vi "XNET Database Export.vi"(0 "cluster in":refnum<k21>, 5 "filepath":path, 11 "error in (no error)":errorcluster) -> (4 "cluster out":refnum<k21>, 15 "error out":errorcluster)   [LabVIEW 2018]
doc: "Exports the cluster to a file in a specific format (.dbc for a CAN cluster, .ldf for a LIN cluster)."
uses:
  nixlvapi.dll
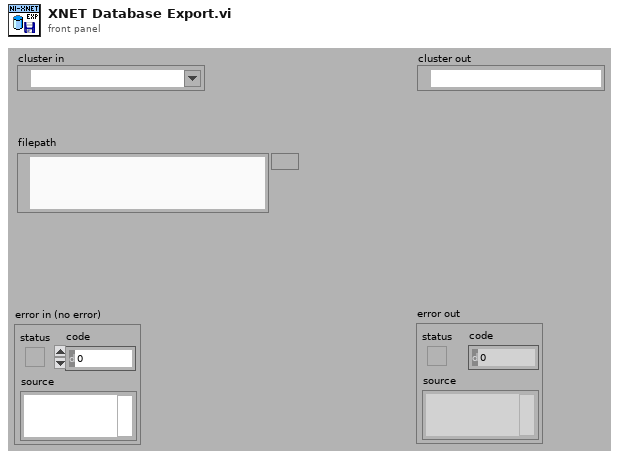
[diagram p1: front panel]
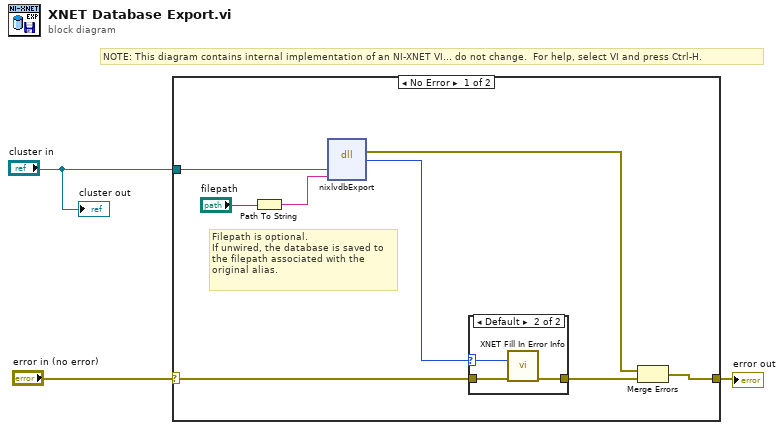
[diagram p0: block diagram]
diagram:
  # "NOTE: This diagram contains internal implementation of an NI-XNET VI... do not change.  For help, select VI and press Ctrl-H."
  n1 = case shown="No Error" "error in (no error)" {
    selector: "error in (no error)" -> [w8 w16]
    tunnel: "cluster in" -> [w11 _]
    tunnel: [w5 w16] -> w3
    frame No Error {
      # "Filepath is optional.\nIf unwired, the database is saved to\nthe filepath associated with the\noriginal alias."
      n2 = Path To String(path="filepath") -> (string=w9:string)
      n3 = dll-call lib="nixlvapi.*" fn="nixlvdbExport" ("nilvxaiu.dll:lvxenDatabaseSave")("reference"=w11, "filepath"=w9) -> (error out=w4:errorcluster, "return type"=w6:i32)  [unwired: 4 in, 2 out]
      n4 = case shown="Default" w6 {
        selector: w6 -> [_ w13]
        tunnel: w8 -> [w12 w14]
        tunnel: [w12 w15] -> w7
        frame 0 {
        }
        frame Default {
          n5 = call "XNET Fill In Error Info.vi"("status code"=w13, "error in"=w14) -> ("error out"=w15:errorcluster)  [unwired: 13 out]
        }
      }
      n6 = Merge Errors(w4, w7) -> (w5:errorcluster)
    }
    frame Error {
    }
  }
  "error out" <- w3
  "cluster out" <- "cluster in"
